vi "Update ChartArea.vi"(8 "error in (no error)":errorcluster, 10 "ChartArea":T1={"Background"={"Color"={"Color"=0, "alpha"=76}, "HatchStyle"=0, "GradientStyle"=0}, "Border"={"DashStyle"=enum."NotSet", "color"={"Color"=0, "alpha"=76}, "Width"=2}, "3D"={"Enable 3D"=FALSE, "LightStyle"=enum."None", "WallWidth"=0, "Perspective"=0, "PointDepth"=0, "PointGapDepth"=0}} {"Border"."color"."alpha" scale=0.0..255.0; "Background"."GradientStyle" items=["None", "LeftRight", "TopBottom", "Center", "DiagonalLeft", "DiagonalRight", "HorizontalCenter", "VerticalCenter"]; "Background"."HatchStyle" items=["None", "BackwardDiagonal", "Cross", "DarkDownwardDiagonal", "DarkHorizontal", "DarkUpwardDiagonal", "DarkVertical", "DashedDownwardDiagonal", "DashedHorizontal", "DashedUpwardDiagonal", "DashedVertical", "DiagonalBrick", "DiagonalCross", "Divot", "DottedDiamond", "DottedGrid", "ForwardDiagonal", "Horizontal", "HorizontalBrick", "LargeCheckerBoard", "LargeConfetti", "LargeGrid", "LightDownwardDiagonal", "LightHorizontal", "LightUpwardDiagonal", "LightVertical", "NarrowHorizontal", "NarrowVertical", "OutlinedDiamond", "Percent05", "Percent10", "Percent20", "Percent25", "Percent30", "Percent40", "Percent50", "Percent60", "Percent70", "Percent75", "Percent80", "Percent90", "Plaid", "Shingle", "SmallCheckerBoard", "SmallConfetti", "SmallGrid", "SolidDiamond", "Sphere", "Trellis", "Vertical", "Wave", "Weave", "WideDownwardDiagonal", "WideUpwardDiagonal", "ZigZag"]; "Background"."Color"."alpha" scale=0.0..255.0}, 11 ".NET Refnum in":refnum<k24>) -> (0 "error out":errorcluster, 3 ".NET Refnum out":refnum<k24>)   [LabVIEW 2014, in "XMSChart.xctl"]
uses:
  XMSChart.xctl
  System.Windows.Forms.DataVisualization
  Controls/ChartArea.ctl
  Controls/Background.ctl
  Controls/Color.ctl
  Controls/Border.ctl
  Controls/3D.ctl
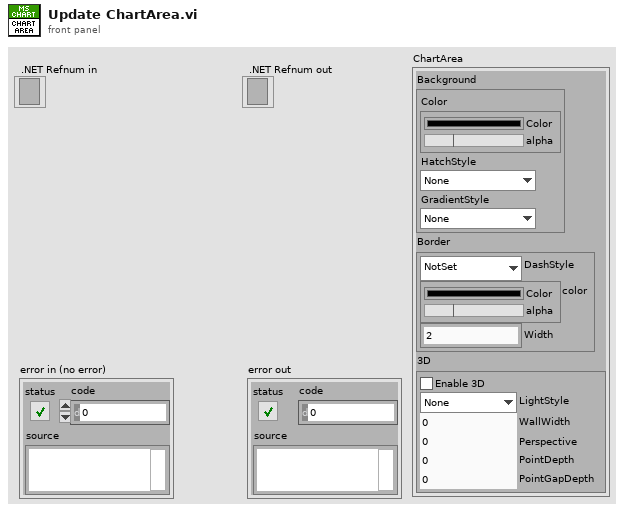
[diagram p1: front panel]
types:
  T1 = typedef "XMSChart.xctl/ChartArea.ctl" = cluster{"Background":T2, "Border":T4, "3D":T5}
  T2 = typedef "XMSChart.xctl/Background.ctl" = cluster{"Color":T3, "HatchStyle":i32, "GradientStyle":i32}
  T3 = typedef "XMSChart.xctl/Color.ctl" = cluster{"Color":u32, "alpha":u8}
  T4 = typedef "XMSChart.xctl/Border.ctl" = cluster{"DashStyle":enum16{"NotSet", "Dash", "DashDot", "DashDotDot", "Dot", "Solid"}, "color":T3, "Width":i32}
  T5 = typedef "XMSChart.xctl/3D.ctl" = cluster{"Enable 3D":bool, "LightStyle":enum16{"None", "Simplistic", "Realistic"}, "WallWidth":i32, "Perspective":i32, "PointDepth":i32, "PointGapDepth":i32}
  T6 = enum16{"NotSet", "Dash", "DashDot", "DashDotDot", "Dot", "Solid"}
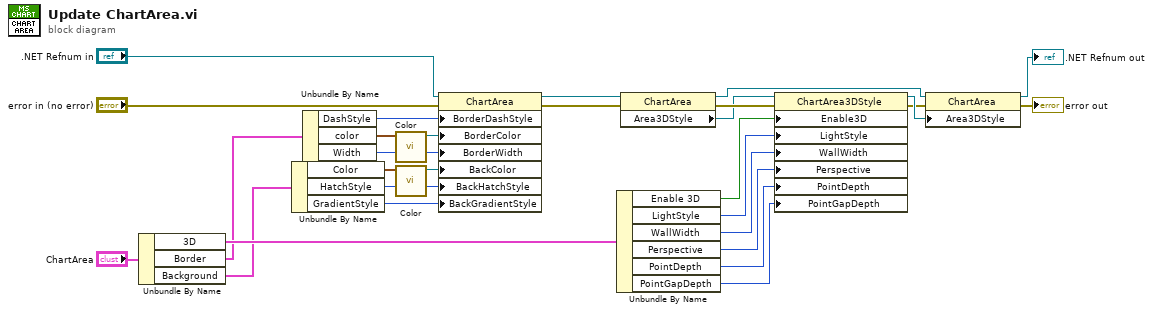
[diagram p0: block diagram]
diagram:
  n1 = Unbundle By Name("ChartArea") -> ("3D"=w29:T5, "Border"=w11:T4, "Background"=w6:T2)
  n2 = Unbundle By Name(w6) -> ("Color"=w5:T3, "HatchStyle"=w3:i32, "GradientStyle"=w2:i32)
  n3 = Unbundle By Name(w11) -> ("DashStyle"=w7:T6, "color"=w10:T3, "Width"=w9:i32)
  n4 = call "Color.vi"("BGK Color"=w10) -> (".NET Refnum out"=w8:refnum<k24>)  [unwired: 10 in]
  n5 = call "Color.vi"("BGK Color"=w5) -> (".NET Refnum out"=w4:refnum<k24>)  [unwired: 10 in]
  n6 = property on="Property Node" class="ChartArea"(reference=".NET Refnum in", error in="error in (no error)", "BorderDashStyle"=w7, "BorderColor"=w8, "BorderWidth"=w9, "BackColor"=w4, "BackHatchStyle"=w3, "BackGradientStyle"=w2) -> (reference out=w27:refnum<k24>, error out=w1:errorcluster)
  n7 = Unbundle By Name(w29) -> ("Enable 3D"=w12:bool, "LightStyle"=w13:enum16{"None", "Simplistic", "Realistic"}, "WallWidth"=w14:i32, "Perspective"=w15:i32, "PointDepth"=w16:i32, "PointGapDepth"=w17:i32)
  n8 = property on="Property Node" class="ChartArea"(reference=w27, error in=w1) -> (reference out=w24:refnum<k24>, error out=w23:errorcluster, "Area3DStyle"=w22:refnum<k24>)
  n9 = property on="Property Node" class="ChartArea3DStyle"(reference=w22, error in=w23, "Enable3D"=w12, "LightStyle"=w13, "WallWidth"=w14, "Perspective"=w15, "PointDepth"=w16, "PointGapDepth"=w17) -> (reference out=w19:refnum<k24>, error out=w18:errorcluster)
  n10 = property on="Property Node" class="ChartArea"(reference=w24, error in=w18, "Area3DStyle"=w19) -> (reference out=→".NET Refnum out":refnum<k24>, error out=→"error out":errorcluster)
